vi "Set Loaded Instrument Configuration.vi"(8 "Error In":errorcluster, 9 "Config from JSON":refnum<class "Config from JSON.lvclass">, 10 "Instrument Identifier":string) -> (0 "Error Out":errorcluster)   [LabVIEW 2019, in "Instrument Manager.lvclass"]
uses:
  Instrument Manager.lvclass
  Instrument Manager.lvclass/Instrument Manager.ctl
  Config from JSON/Config from JSON.lvclass
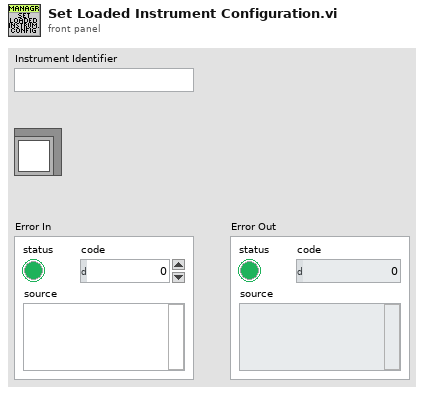
[diagram p1: front panel]
types:
  T1 = typedef "Instrument Manager.lvclass/ObjectAttributes.ctl" = cluster{"ICreate Action Point":refnum<class "ICreate Action Point.lvclass">, "IInstruments":map{string, refnum<class "IInstrument.lvclass">}, "IVirtual Instruments":map{string, refnum<class "IVirtual Instrument.lvclass">}, "Instrument Configurations":map{string, refnum<class "Config from JSON.lvclass">}, "Virtual Instrument Configurations":map{string, refnum<class "Config from JSON.lvclass">}, "Action Point Configurations":map{string, refnum<class "Config from JSON.lvclass">}, "Action Points":map{string, refnum<class "Action Point.lvclass">}}
  T2 = map{string, refnum<class "Config from JSON.lvclass">}
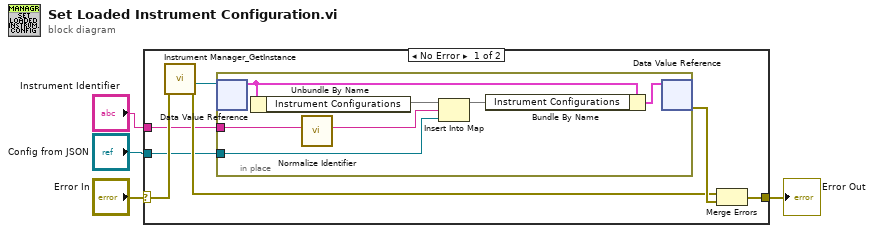
[diagram p0: block diagram]
diagram:
  n1 = case shown="No Error" "Error In" {
    selector: "Error In" -> [w11 w19]
    tunnel: [w8 w19] -> w3
    tunnel: "Config from JSON" -> [w6 _]
    tunnel: "Instrument Identifier" -> [w5 _]
    frame No Error {
      n2 = call "Instrument Manager_GetInstance.vi"("Error In"=w11) -> ("Error Out"=w9:errorcluster, "DVRRefOut"=w7:refnum<data-value>)  [unwired: 6 in, 3 out]
      n3 = in-place {
        in-place-border: w6 -> [w14]
        in-place-border: w5 -> [w15]
        n4 = in-place-dvr #1(w7) -> (w17:T1)  [unwired: 1 out]
        n5 = Unbundle By Name(w17) -> ("Instrument Configurations"=w16:T2)
        n6 = call "Normalize Identifier.vi"("Identifier"=w15) -> ("Normalized Identifier"=w12:string)  [unwired: 10 in]
        n7 = Insert Into Map(map in=w16, key=w12, value=w14) -> (map out=w13:T2)  [unwired: 2 out]
        n8 = Bundle By Name(cluster=w17, "Instrument Configurations"=w13) -> (w18:T1)
        n9 = in-place-dvr #1(w18) -> (w10:errorcluster)  [unwired: 1 out]
      }
      n10 = Merge Errors(w9, w10) -> (w8:errorcluster)
    }
    frame Error {
    }
  }
  "Error Out" <- w3
